vi "PTestbed_Cycling.vi"() -> ()   [LabVIEW 2020]
panel:
  out "DAQ error out":errorcluster[](array[cluster])
  out "PS error out":errorcluster[](array[cluster])
  in  "Battery Select":T1(ring)
  in  "Current Cutoff":dbl
  in  "Number of Cycles":i32
  in  "Charge filepath":path
  in  "Discharge filepath":path
  in  "Testname":string
  in  "Starting Cycle":i32
  in  "Wait time":dbl
  in  "Discharge Current Setpoint":dbl format="%#.6g"
  in  "Charge Current Setpoint":dbl format="%#.6g"
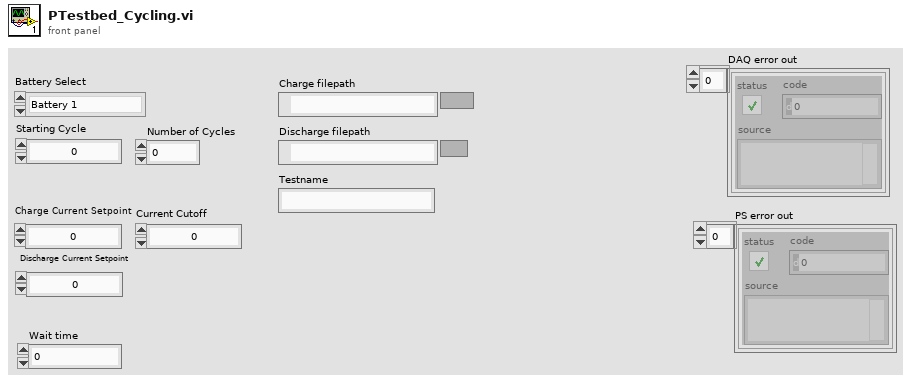
[diagram p1: front panel]
types:
  T1 = enum16{"Battery 1", "Battery 2", "Battery 3", "Battery 1&2", "Battery 1&3", "Battery 2&3", "Battery 1&2&3"}
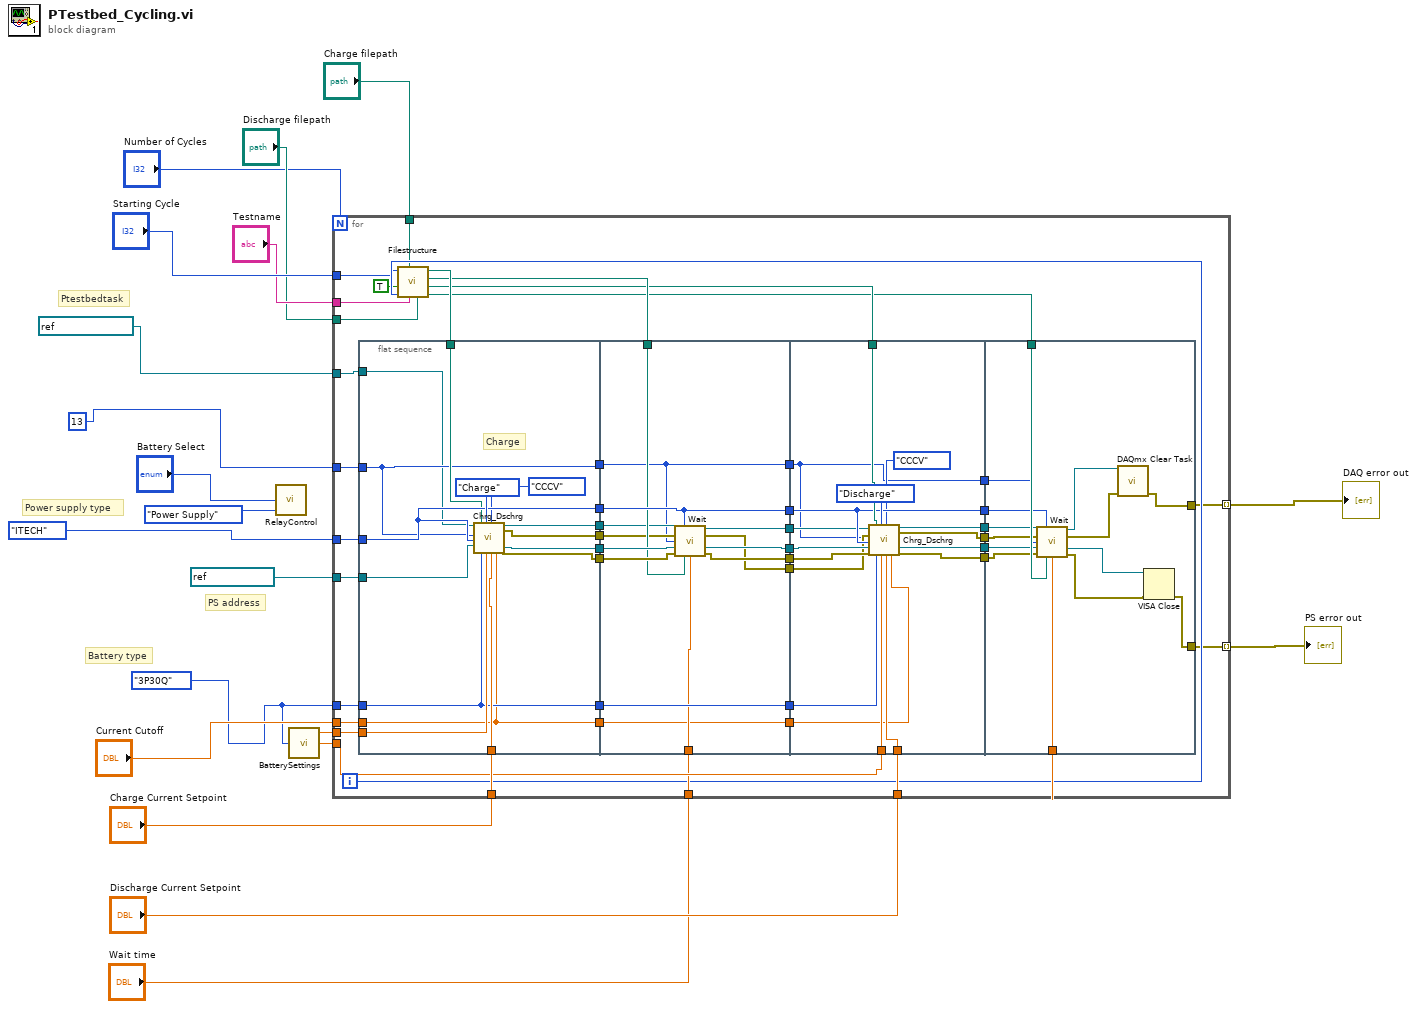
[diagram p0: block diagram]
diagram:
  w1 = enum16{"30Q", "40T", "2P30Q", "3P30Q"}."3P30Q" ("Battery Type")
  # "Battery type"
  # "PS address"
  # "Power supply type"
  # "Ptestbedtask"
  n1 = call "RelayControl.vi"("NHR or Battery Analyzer"=enum16{"Battery Analyzer", "Power Supply"}."Power Supply", "Battery Select"="Battery Select") -> ()  [unwired: 3 in]
  n2 = call "BatterySettings.vi"("Battery Type"=w1) -> ("Min Voltage (V)"=w18:dbl, "Max Voltage (V)"=w20:dbl)  [unwired: 2 in, 1 out]
  n3 = for {
    N: "Number of Cycles" -> [_]
    tunnel: 13 ("#DAQ outputs (1-13)") -> [w52]
    tunnel: enum16{"NHR", "ITECH"}."ITECH" ("PS type") -> [w51]
    tunnel: w20 -> [w50]
    tunnel: w1 -> [w49]
    tunnel: "Charge Current Setpoint" -> [w48]
    tunnel: w18 -> [w47]
    tunnel: "Discharge Current Setpoint" -> [w46]
    tunnel: "Wait time" -> [w41]
    tunnel: "Starting Cycle" -> [w39]
    tunnel: "Testname" -> [w37]
    tunnel: "Discharge filepath" -> [w36]
    tunnel: "Charge filepath" -> [w35]
    tunnel: "Current Cutoff" -> [w34]
    tunnel: [w24] -> w6 mode=indexing
    tunnel: [w23] -> w5 mode=indexing
    tunnel: refnum<k21> "PTesbedTask" ("Data Task in") -> [w22]
    tunnel: refnum<visa-resource-name> "ITECH-PS3" ("PS Visa Out") -> [w21]
    i -> [w40]
    n4 = flat-sequence {
      tunnel: w22 -> [w71]
      tunnel: w52 -> [w72]
      tunnel: w51 -> [w75]
      tunnel: w49 -> [w74]
      tunnel: w50 -> [w79]
      tunnel: w48 -> [w78]
      tunnel: [w77] -> w65
      tunnel: [w76] -> w64
      tunnel: [w75] -> w63
      tunnel: [w72] -> w62
      tunnel: [w74] -> w61
      tunnel: w45 -> [w73]
      tunnel: w34 -> [w69]
      tunnel: [w69] -> w33
      tunnel: [w68] -> w31
      tunnel: [w67] -> w30
      tunnel: w21 -> [w66]
      tunnel: w65 -> [w94]
      tunnel: w64 -> [w93]
      tunnel: w63 -> [w90]
      tunnel: [w92] -> w60
      tunnel: [w91] -> w59
      tunnel: w62 -> [w81]
      tunnel: [w81] -> w58
      tunnel: [w90] -> w57
      tunnel: w61 -> [w89]
      tunnel: [w89] -> w56
      tunnel: w44 -> [w88]
      tunnel: w41 -> [w87]
      tunnel: w33 -> [w86]
      tunnel: [w86] -> w32
      tunnel: w31 -> [w85]
      tunnel: w30 -> [w84]
      tunnel: [w83] -> w29
      tunnel: [w82] -> w28
      tunnel: w60 -> [w111]
      tunnel: w59 -> [w110]
      tunnel: w58 -> [w95]
      tunnel: w57 -> [w102]
      tunnel: w56 -> [w109]
      tunnel: w47 -> [w108]
      tunnel: w46 -> [w107]
      tunnel: w43 -> [w105]
      tunnel: [w104] -> w55
      tunnel: [w103] -> w54
      tunnel: [w102] -> w53
      tunnel: w32 -> [w100]
      tunnel: w29 -> [w99]
      tunnel: w28 -> [w98]
      tunnel: [w97] -> w27
      tunnel: [w96] -> w26
      tunnel: [w95] -> w25
      tunnel: w42 -> [w125]
      tunnel: w55 -> [w124]
      tunnel: w54 -> [w123]
      tunnel: w41 -> [w122]
      tunnel: w53 -> [w121]
      tunnel: [w114] -> w24
      tunnel: w27 -> [w120]
      tunnel: w26 -> [w119]
      tunnel: [w115] -> w23
      tunnel: w25 -> [w118]
      frame #0 {
        # "Charge"
        n5 = call "Chrg_Dschrg.vi"("Data Task in"=w71, "#DAQ outputs (1-13)"=w72, "PS type"=w75, "PS VISA in"=w66, "DischargeCyclePath"=w73, "Battery Type"=w74, "Charge/discharge"=enum8{"Charge", "Discharge"}."Charge", "Charge/Discharge Voltage Setpoint"=w79, "CC or CCCV"=enum16{"CC", "CCCV"}."CCCV", "Current Setpoint"=w78, "Current Cutoff"=w69) -> ("data task out"=w68:refnum<k21>, "data task error out"=w67:errorcluster, "PS VIS resource name out"=w77:refnum<visa-resource-name>, "PS error out"=w76:errorcluster)  [unwired: 5 in]
      }
      frame #1 {
        n6 = call "Wait.vi"("Data Task in"=w85, "PS type"=w90, "data task error in"=w84, "#DAQ outputs (1-13)"=w81, "PS VISA in"=w94, "PS error in"=w93, "Wait Filepath"=w88, "Wait time"=w87) -> ("data task out"=w83:refnum<k21>, "data task error out"=w82:errorcluster, "PS Visa Out"=w92:refnum<visa-resource-name>, "PS error out"=w91:errorcluster)  [unwired: 4 in]
      }
      frame #2 {
        n7 = call "Chrg_Dschrg.vi"("Data Task in"=w99, "data task error in"=w98, "#DAQ outputs (1-13)"=w95, "PS type"=w102, "PS VISA in"=w111, "PS error in"=w110, "DischargeCyclePath"=w105, "Battery Type"=w109, "Charge/discharge"=enum8{"Charge", "Discharge"}."Discharge", "Charge/Discharge Voltage Setpoint"=w108, "CC or CCCV"=enum16{"CC", "CCCV"}."CCCV", "Current Setpoint"=w107, "Current Cutoff"=w100) -> ("data task out"=w97:refnum<k21>, "data task error out"=w96:errorcluster, "PS VIS resource name out"=w104:refnum<visa-resource-name>, "PS error out"=w103:errorcluster)  [unwired: 3 in]
      }
      frame #3 {
        n8 = call "Wait.vi"("Data Task in"=w120, "PS type"=w121, "data task error in"=w119, "#DAQ outputs (1-13)"=w118, "PS VISA in"=w124, "PS error in"=w123, "Wait Filepath"=w125, "Wait time"=w122) -> ("data task out"=w117:refnum<k21>, "data task error out"=w116:errorcluster, "PS Visa Out"=w113:refnum<visa-resource-name>, "PS error out"=w112:errorcluster)  [unwired: 4 in]
        n9 = call <vilib>:"DAQmx Clear Task.vi"("task in"=w117, "error in"=w116) -> ("error out"=w115:errorcluster)  [unwired: 13 in]
        n10 = VISA Close(VISA resource name=w113, error in (no error)=w112) -> (error out=w114:errorcluster)
      }
    }
    n11 = call "Filestructure.vi"("Discharge filepath"=w36, "Batteryname"=w37, "Charge filepath"=w35, "For loop i"=w40, "In for loop"=TRUE, "Starting Cycle"=w39) -> ("DischargeWaitPath"=w42:path, "DischargeCyclePath"=w43:path, "ChargeWaitPath"=w44:path, "ChargeCyclePath"=w45:path)  [unwired: 1 in, 1 out]
  }
  "PS error out" <- w6
  "DAQ error out" <- w5
